vi "Make Python Array.vi"(1 "Pythonic Values":string[](array[string])) -> (0 "Pythonic Array":string)   [LabVIEW 2016, in "OPI.lvclass"]
uses:
  OPI.lvclass
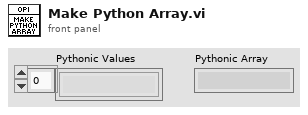
[diagram p1: front panel]
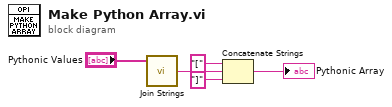
[diagram p0: block diagram]
diagram:
  n1 = call <vilib>:"Join Strings.vi"("Strings In"="Pythonic Values") -> ("String"=w5:string)  [unwired: 2 in]
  n2 = Concatenate Strings("[" ("string"), w5, "]" ("string")) -> (→"Pythonic Array":string)
